vi "UnwrapPhaseNegative.vi"(11 "radian":dbl[](array[numeric])) -> (3 "degrees":dbl[](array[numeric]))   [LabVIEW 2017, in "McsaAnalysisLowRate.lvlib"]
uses:
  <vilib>/addons/InsightCM/Devices/Shared/Mcsa/McsaAnalysisLowRate/McsaAnalysisLowRate.lvlib
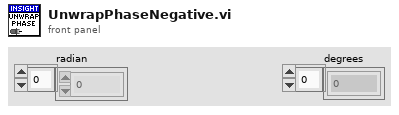
[diagram p1: front panel]
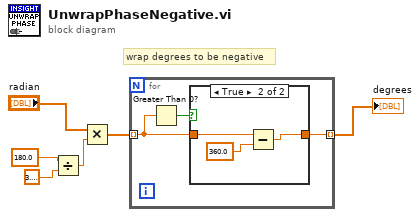
[diagram p0: block diagram]
diagram:
  # "wrap degrees to be negative"
  n1 = Divide(x=180.0, y=3.141592653589793) -> (x/y=w4:dbl)
  n2 = Multiply(x="radian", y=w4) -> (x*y=w1:dbl[])
  n3 = for {
    tunnel: w1 -> [w8] mode=indexing
    tunnel: [w7] -> w6 mode=indexing
    n4 = Greater Than 0?(x=w8) -> (x > 0?=w9:bool)
    n5 = case shown="True" w9 {
      tunnel: w8 -> [w10 w12]
      tunnel: [w10 w11] -> w7
      frame False {
      }
      frame True {
        n6 = Subtract(x=w12, y=360.0) -> (x-y=w11:dbl)
      }
    }
  }
  "degrees" <- w6
